vi "Excel Write.vi"(8 "error in (no error)":errorcluster caption="错误输入（无错误）", 10 "Write":string[][](array[string]), 11 "Path":path=path "E:/AgainDo/项目/进行中/莱茵化学FCM报价系统/FCM 2021.08.26/Document/材料管理文件.xlsx") -> (0 "error out":errorcluster caption="错误输出")   [LabVIEW 2020]
uses:
  <vilib>/Utility/NIReport.llb/Report Type.ctl
  <vilib>/Utility/NIReport.llb/Append Text Table to Report (wrap).vi
  <vilib>/Utility/NIReport.llb/NI_report.lvclass
  <vilib>/Utility/NIReport.llb/NI_ReportGenerationCore.lvlib
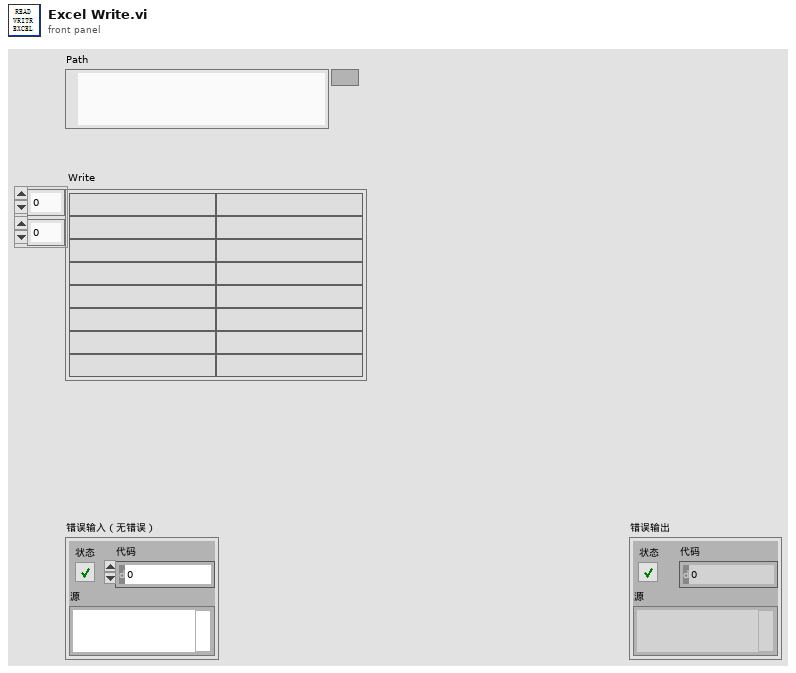
[diagram p1: front panel]
types:
  T1 = enum16{"maximized", "minimized", "normal", "no change"}
  T2 = typedef "NI_ReportGenerationCore.lvlib/Report Type.ctl" = enum16{"HTML", "Word", "Excel"}
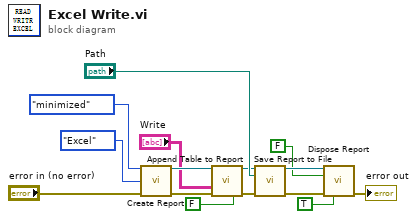
[diagram p0: block diagram]
diagram:
  n1 = call <vilib>:"Create Report.vi"("window state (normal)"=T1."minimized", "report type"=Report_Type."Excel", "error in (no error)"="error in (no error)") -> ("report out"=w10:refnum<class "NI_report.lvclass">, "error out"=w9:errorcluster)  [unwired: 11 in]
  n2 = call-poly <vilib>:"Append Table to Report.vi"("report in"=w10, "text data"="Write", "error in (no error)"=w9, "show grid lines (YES)"=FALSE) -> ("report out"=w5:refnum<class "NI_report.lvclass">, "error out"=w6:errorcluster)  [unwired: 8 in, 2 out]
  n3 = call-dynamic "Save Report to File.vi"("report in"=w5, "report file path"="Path", "error in (no error)"=w6) -> ("report out"=w7:refnum<class "NI_report.lvclass">, "error out"=w8:errorcluster)  [unwired: 11 in]
  n4 = call-dynamic "Dispose Report.vi"("report in"=w7, "wait until printing completed? (T)"=FALSE, "error in (no error)"=w8, "close report? (T)"=TRUE) -> ("error out"=→"error out":errorcluster)  [unwired: 11 in]
